vi "Write Interface string cluster.vi"(10 "Interface sting cluster":T1={"Interface"="", "IDN string"="", "Instance"=1}, 11 "Instrument in":refnum<class "Instrument.lvclass">) -> (3 "Instrument out":refnum<class "Instrument.lvclass">)   [LabVIEW 2020, in "Instrument.lvclass"]
uses:
  Instrument.lvclass
  Controls/Interface String Cluster.ctl
  Instrument.lvclass/Instrument.ctl
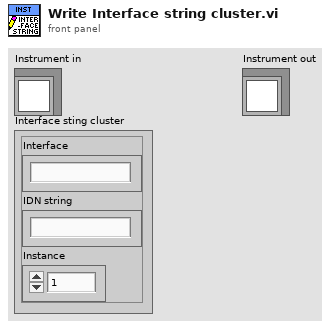
[diagram p1: front panel]
types:
  T1 = typedef "Instrument.lvclass/Interface String Cluster.ctl" = cluster{"Interface":string, "IDN string":string, "Instance":i32}
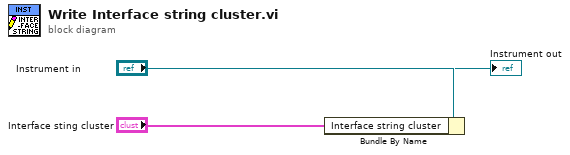
[diagram p0: block diagram]
diagram:
  n1 = Bundle By Name(cluster="Instrument in", "Interface string cluster"="Interface sting cluster") -> (→"Instrument out":refnum<class "Instrument.lvclass">)
